vi "leds_on_off.vi"(0 "error in":errorcluster, 2 "Cluster":T1, 3 "node":string) -> (1 "error out":errorcluster)   [LabVIEW 2015]
uses:
  ROS/Code/Console/Servers/ServerSubs/TopicDef.ctl
  ROS/Code/SubVIs/_ROSDirection.ctl
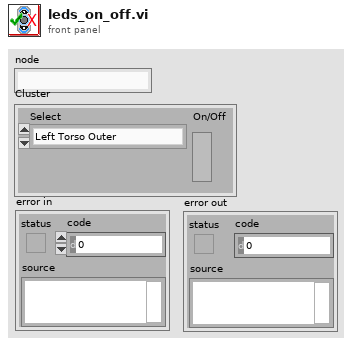
[diagram p1: front panel]
types:
  T1 = cluster{"Select":enum16{"Left Torso Outer", "Left Torso Inner", "Right Torso Outer", "Right Torso Inner", "Left Arm Outer", "Right Arm Outer", "Right Arm Inner", "Left Arm Inner"}, "On/Off":bool}
  T2 = typedef "TopicDef.ctl" = cluster{"Topic":string, "Type":string, "Action":T3, "Update (ms)":u16, "queue size":u16}
  T3 = typedef "_ROSDirection.ctl" = enum16{"Node", "Publisher", "Subscriber", "ServiceClient", "ServiceProvider"}
  T4 = enum16{"Left Torso Outer", "Left Torso Inner", "Right Torso Outer", "Right Torso Inner", "Left Arm Outer", "Right Arm Outer", "Right Arm Inner", "Left Arm Inner"}
  T5 = typedef "_ROSControl.ctl" = cluster{"topic port":u16, "Node":string, "topic":string, "type":string, "node port":u16, "error ":errorcluster, "Direction":T3, "Update (ms)":u16, "FIFO size":u16}
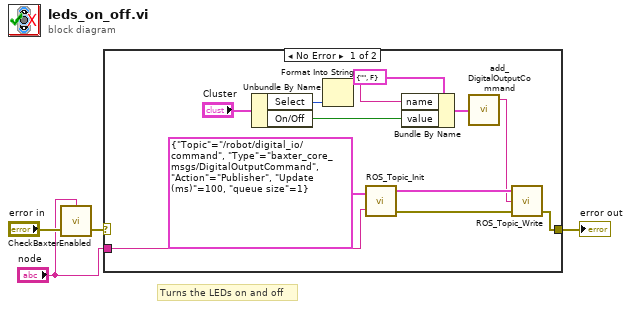
[diagram p0: block diagram]
diagram:
  # "Turns the LEDs on and off"
  n1 = call "CheckBaxterEnabled.vi"("error in"="error in", "node"="node") -> ("error out"=w3:errorcluster)  [unwired: 2 in]
  n2 = case shown="No Error" w3 {
    selector: w3 -> [_ w17]
    tunnel: "node" -> [w14 _]
    tunnel: [w8 w17] -> w1
    frame No Error {
      n3 = Unbundle By Name("Cluster") -> ("Select"=w6:T4, "On/Off"=w5:bool)
      n4 = Format Into String(w6) -> (resulting string=w11:string)  [unwired: 3 in, 1 out]
      n5 = call "ROS_Topic_Init.vi"("Definitions"=T2 {"Topic"="/robot/digital_io/command", "Type"="baxter_core_msgs/DigitalOutputCommand", "Action"=enum."Publisher", "Update (ms)"=100, "queue size"=1}, "node"=w14) -> ("ROS out"=w15:T5, "error out"=w13:errorcluster)  [unwired: 1 in]
      n6 = Bundle By Name(cluster=cluster{"name":string, "value":bool} {"name"="", "value"=FALSE}, "name"=w11, "value"=w5) -> (w10:cluster{"name":string, "value":bool})
      n7 = call "add_DigitalOutputCommand.vi"("Digital Output Command"=w10) -> ("msg out"=w9:string)  [unwired: 4 in]
      n8 = call "ROS_Topic_Write.vi"("error in (no error)"=w13, "Msg in"=w9, "ROS in"=w15) -> ("error out"=w8:errorcluster)  [unwired: 1 in, 1 out]
    }
    frame Error {
    }
  }
  "error out" <- w1
